vi "ex_4_8_inaczej.vi"() -> ()   [LabVIEW 2020]
panel:
  out "Array":u32[][](array[numeric])
  in  "M":i32
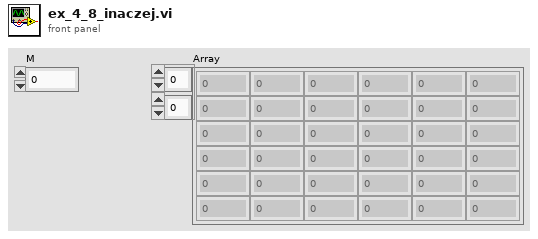
[diagram p1: front panel]
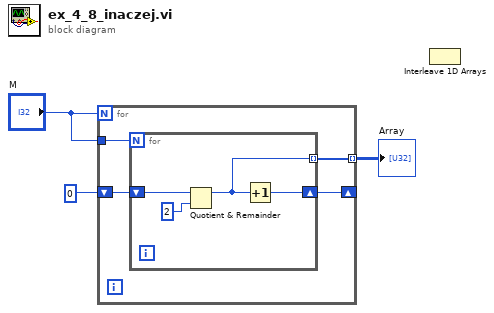
[diagram p0: block diagram]
diagram:
  n1 = for {
    N: "M" -> [_]
    tunnel: "M" -> [w7]
    tunnel: [w6] -> w2 mode=indexing
    shift-right: [w4] -> _
    shift-left: u32 0 -> [w5]
    n2 = for {
      N: w7 -> [_]
      tunnel: [w8] -> w6 mode=indexing
      shift-right: [w9] -> w4
      shift-left: w5 -> [w10]
      n3 = Quotient & Remainder(x=w10, y=u32 2) -> (x-y*floor(x/y)=w8:u32)  [unwired: 1 out]
      n4 = Increment(x=w8) -> (x+1=w9:u32)
    }
  }
  "Array" <- w2
  n5 = Interleave 1D Arrays() -> ()  [unwired: 2 in, 1 out]
